vi "Listen and Acknowledge Commands.vi"() -> ()   [LabVIEW 2013]
doc: "This example demostrates how to use UDP with STM to broadcast messages to multiple systems at once.\n\nThe \"Listen and Acknowledge Commands\" VI must be started first."
uses:
  vi.lib/NI/STM/UDP/UDP Read Options.ctl
  vi.lib/NI/STM/UDP/Read Meta Data (UDP Ref).vi
  vi.lib/NI/STM/UDP/Get Connection Reference (UDP).vi
  vi.lib/NI/STM/UDP/Read Meta Data (UDP Clst).vi
  vi.lib/NI/STM/UDP/Read Message (UDP).vi
  vi.lib/NI/STM/UDP/Write Message (UDP).vi
  vi.lib/NI/STM/NI STM.lvlib
panel:
  out "error out":errorcluster
  out "Last Command":string
  in  "remote port":u16=61556
  in  "stop":bool
  in  "local port":u16=61557
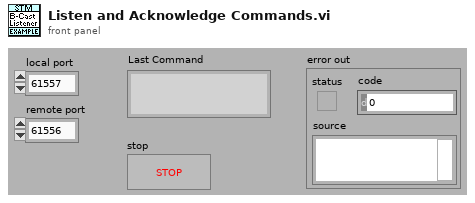
[diagram p1: front panel]
types:
  T1 = typedef "NI STM.lvlib/UDP Read Options.ctl" = cluster{"ignore timeout error":bool, "timeout ms (1000)":i32, "max size (548)":i32}
  T2 = typedef "NI STM.lvlib/UDP Connection Info.ctl" = cluster{"connection ID":refnum<k16>, "meta data":T3[]}
  T3 = typedef "NI STM.lvlib/MetaDataElement.ctl" = string
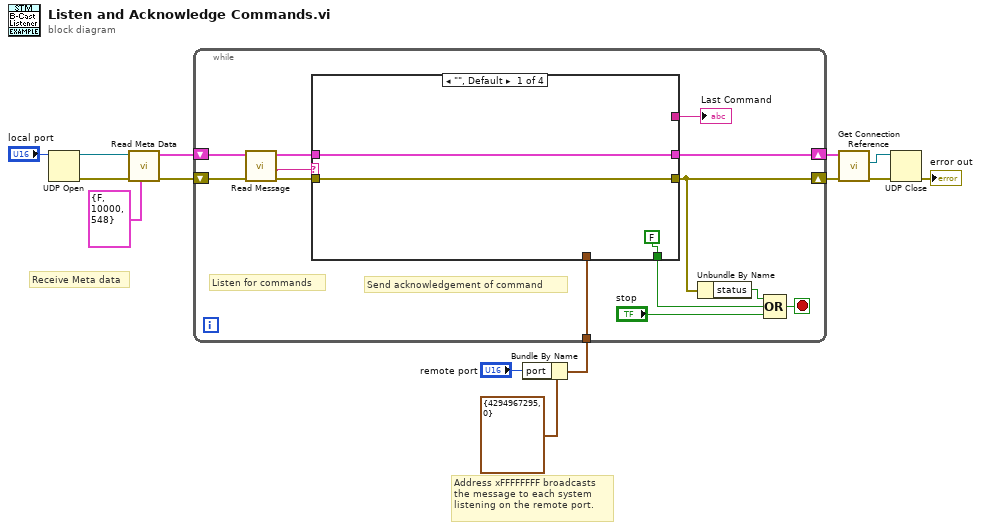
[diagram p0: block diagram]
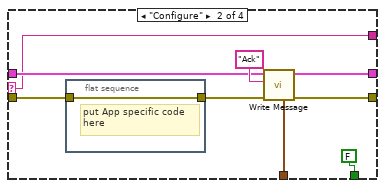
[diagram p2: hidden frame]
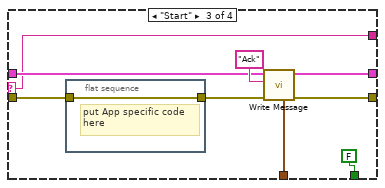
[diagram p3: hidden frame]
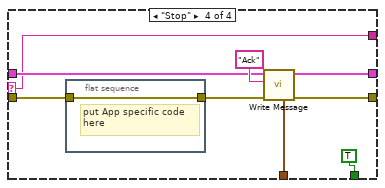
[diagram p4: hidden frame]
diagram:
  # "Address xFFFFFFFF broadcasts\nthe message to each system\nlistening on the remote port."
  # "Receive Meta data"
  n1 = UDP Open(11:"local port") -> (port=w14:refnum<k16>, 0:w13:errorcluster)  [unwired: 1 in, 4 out]
  n2 = call-poly "Read Meta Data.vi"("options"=T1 {"ignore timeout error"=FALSE, "timeout ms (1000)"=10000, "max size (548)"=548} ("Options"), "error in"=w13, "connection ID"=w14) -> ("error out"=w10:errorcluster, "connection info out"=w11:T2)  [unwired: 7 out]
  n3 = Bundle By Name(cluster=cluster{"address":u32, "port":u16} {"address"=4294967295, "port"=0} ("Address"), "port"="remote port") -> (w2:cluster{"address":u32, "port":u16})
  n4 = while {
    shift-right: [w23] -> w7
    shift-left: w11 -> [w27]
    shift-right: [w16] -> w8
    shift-left: w10 -> [w26]
    tunnel: w2 -> [w17]
    stop <- w21 stop-if-true
    # "Send acknowledgement of command"
    # "Listen for commands"
    n5 = call-poly "Read Message.vi"("error in"=w26, "connection info in"=w27) -> ("error out"=w25:errorcluster, "name"=w18:T3, "connection info out"=w24:T2)  [unwired: 1 in, 6 out]
    n6 = case shown="\"\", Default" w18 {
      selector: w18 -> [_ w32 w42 w52]
      tunnel: w25 -> [w29 w36 w46 w56]
      tunnel: w24 -> [w30 w33 w43 w53]
      tunnel: [w30 w38 w48 w58] -> w23
      tunnel: [w29 w37 w47 w57] -> w16
      tunnel: [_ w32 w42 w52] -> w22
      tunnel: [FALSE FALSE FALSE TRUE] -> w19
      tunnel: w17 -> [_ w31 w41 w51]
      frame "", Default {
      }
      frame "Configure" {
        n7 = flat-sequence {
          tunnel: w36 -> [w40]
          tunnel: [w40] -> w35
          frame #0 {
            # "put App specific code\nhere"
          }
        }
        n8 = call-poly "Write Message.vi"("address"=w31, "error in"=w35, "name"="Ack" ("Name"), "connection info in"=w33) -> ("error out"=w37:errorcluster, "connection info out"=w38:T2)  [unwired: 3 in, 3 out]
      }
      frame "Start" {
        n9 = flat-sequence {
          tunnel: w46 -> [w50]
          tunnel: [w50] -> w45
          frame #0 {
            # "put App specific code\nhere"
          }
        }
        n10 = call-poly "Write Message.vi"("address"=w41, "error in"=w45, "name"="Ack" ("Name"), "connection info in"=w43) -> ("error out"=w47:errorcluster, "connection info out"=w48:T2)  [unwired: 3 in, 3 out]
      }
      frame "Stop" {
        n11 = flat-sequence {
          tunnel: w56 -> [w60]
          tunnel: [w60] -> w55
          frame #0 {
            # "put App specific code\nhere"
          }
        }
        n12 = call-poly "Write Message.vi"("address"=w51, "error in"=w55, "name"="Ack" ("Name"), "connection info in"=w53) -> ("error out"=w57:errorcluster, "connection info out"=w58:T2)  [unwired: 3 in, 3 out]
      }
    }
    "Last Command" <- w22
    n13 = Unbundle By Name(w16) -> ("status"=w15:bool)
    n14 = Compound Arithmetic op=OR(w15, w19, "stop") -> (w21:bool)
  }
  n15 = call-poly "Get Connection Reference.vi"("error in"=w8, "connection info in"=w7) -> ("error out"=w5:errorcluster, "connection ID"=w6:refnum<k16>)  [unwired: 8 out]
  n16 = UDP Close(connection ID=w6, 8:w5) -> (error out=→"error out":errorcluster)  [unwired: 1 out]
